vi "SamsungDemo.vi"() -> ()   [LabVIEW 2015]
panel:
  in  "숫자형 2":dbl
  in  "숫자형":dbl
  out "x+y":dbl
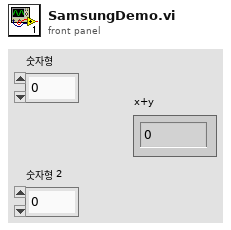
[diagram p1: front panel]
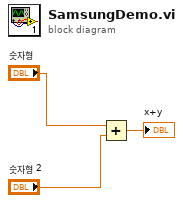
[diagram p0: block diagram]
diagram:
  n1 = Add(x="숫자형", y="숫자형 2") -> (x+y=→"x+y":dbl)
